vi "InputRecorder.vi"(0 "Z Input":dbl, 1 "Y Input":dbl, 2 "X Input":dbl, 3 "Folder":path) -> ()   [LabVIEW 2020]
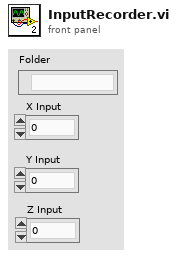
[diagram p1: front panel]
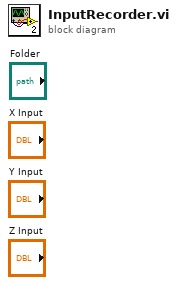
[diagram p0: block diagram]
diagram:
